vi "UIDatabaseAdapter.vi"(8 "error in (no error)":errorcluster, 10 "UI Data In":variant, 11 "UserBasicInfo":refnum<class "UserBasicInfo.lvclass">) -> (0 "error out":errorcluster, 2 "UI Data out":variant, 3 "UserBasicInfo out":refnum<class "UserBasicInfo.lvclass">)   [LabVIEW 2015, in "UserManagement.lvlib" / "UserBasicInfo.lvclass"]
doc: "Functions : <b>this is a adapter to Link database and UI"
uses:
  UserManagement/UserBasicInfo/UserBasicInfo.lvclass
  typedef/Member Basic Info(UI).ctl
  UserManagement/User/typedef/SchoolOfUser.ctl
  UserManagement/User/typedef/GradeOfUser.ctl
  UserManagement/User/typedef/GroupOfUser.ctl
  typedef/Member Basic Info(Database).ctl
  UserManagement/User/User.lvclass
panel:
  out "User Basic Info":T1
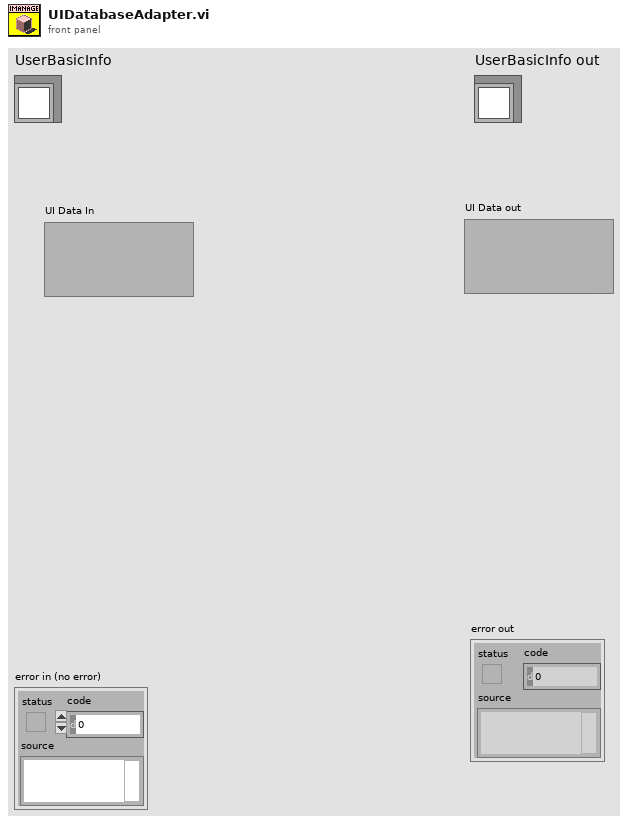
[diagram p1: front panel]
types:
  T1 = typedef "UserManagement.lvlib/UserBasicInfo.lvclass/Member Basic Info(UI).ctl" = cluster{"Name":string, "StudentID":string, "Description":string, "School":T2, "Grade":T3, "Group":T4}
  T2 = typedef "UserManagement.lvlib/User.lvclass/SchoolOfUser.ctl" = enum8{"机电工程学院", "电气工程学院", "航天学院", "能源学院", "理学院", "英才学院"}
  T3 = typedef "UserManagement.lvlib/User.lvclass/GradeOfUser.ctl" = enum16{"大二", "大三", "大四", "研一"}
  T4 = typedef "UserManagement.lvlib/User.lvclass/GroupOfUser.ctl" = enum16{"电控", "机械", "视觉"}
  T5 = typedef "UserManagement.lvlib/UserBasicInfo.lvclass/Member Basic Info(Database).ctl" = cluster{"Name":string, "StudentID":string, "School":string, "Grade":string, "Group":string, "Description":string}
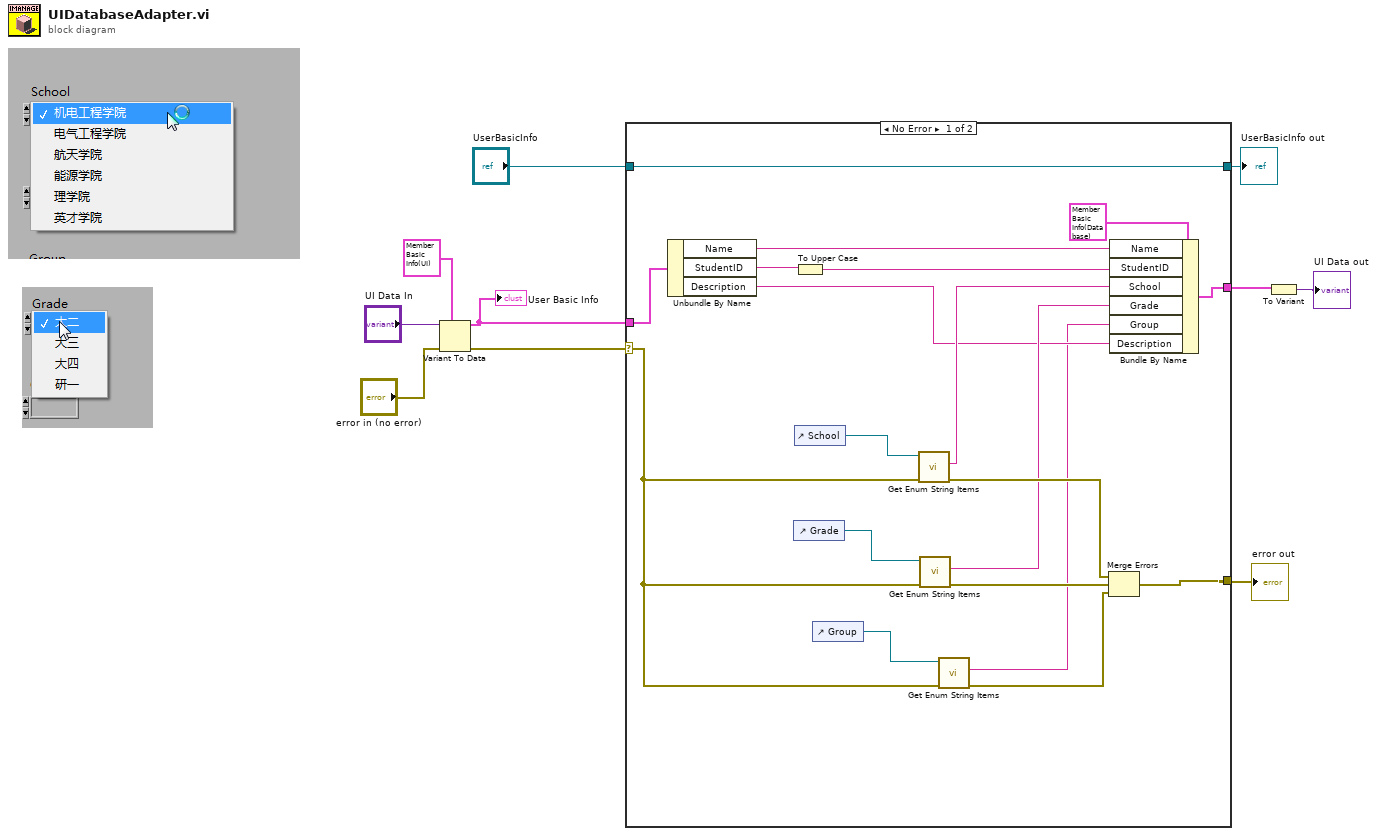
[diagram p0: block diagram]
diagram:
  n1 = Variant To Data(error in="error in (no error)", type=T1 {"Name"="", "StudentID"="", "Description"="", "School"=enum."机电工程学院", "Grade"=enum."大二", "Group"=enum."电控"} ("User Basic Info"), Variant="UI Data In") -> (data=w5:T1, error out=w7:errorcluster)
  "User Basic Info" <- w5
  n2 = case shown="No Error" w7 {
    selector: w7 -> [w13 w31]
    tunnel: [w22 w31] -> w10
    tunnel: [w24 _] -> w4
    tunnel: w5 -> [w17 _]
    tunnel: "UserBasicInfo" -> [w16 w30]
    tunnel: [w16 w30] -> w1
    frame No Error {
      n3 = Unbundle By Name(w17) -> ("Name"=w27:string, "StudentID"=w29:string, "Description"=w15:string)
      n4 = control-ref of="Grade"() -> (w20:refnum<vi>)
      n5 = To Upper Case(1:w29) -> (0:w26:string)
      n6 = control-ref of="School"() -> (w21:refnum<vi>)
      n7 = control-ref of="Group"() -> (w14:refnum<vi>)
      n8 = call "Get Enum String Items.vi"("error in (no error)"=w13, "Enum Refnum"=w21) -> ("error out"=w23:errorcluster, "String"=w25:string)  [unwired: 7 in]
      n9 = call "Get Enum String Items.vi"("error in (no error)"=w13, "Enum Refnum"=w20) -> ("error out"=w18:errorcluster, "String"=w19:string)  [unwired: 7 in]
      n10 = call "Get Enum String Items.vi"("error in (no error)"=w13, "Enum Refnum"=w14) -> ("error out"=w11:errorcluster, "String"=w12:string)  [unwired: 7 in]
      n11 = Merge Errors(w23, w18, w11) -> (w22:errorcluster)
      n12 = Bundle By Name(cluster=T5 {"Name"="姓名", "StudentID"="学号", "School"="学院", "Grade"="年级", "Group"="组别", "Description"="简介"} ("成员基本列表"), "Name"=w27, "StudentID"=w26, "School"=w25, "Grade"=w19, "Group"=w12, "Description"=w15) -> (w24:T5)
    }
    frame Error {
    }
  }
  "error out" <- w10
  "UserBasicInfo out" <- w1
  n13 = To Variant(anything=w4) -> (Variant=→"UI Data out":variant)
